vi "Set Readout Rate and EM Mode.vi"(8 "error in (no error)":errorcluster, 11 "CCDCamera in":refnum<class "CCDCamera.lvclass">) -> (0 "error out":errorcluster, 3 "CCDCamera out":refnum<class "CCDCamera.lvclass">)   [LabVIEW 2018, in "CCDCamera.lvclass"]
uses:
  CCDCamera.lvclass
  C:/Users/observer/Desktop/SPARC4_ACS/SPARC4_ACS/Simulated_CCD_Camera/Simulated_CCD_Camera.lvclass
  Simulated_CCD_Camera/Simulated_CCD_Camera.lvclass/Simulated_CCD_Camera.ctl
  Interface/Interface.lvclass/Interface.ctl
  Interface/Interface.lvclass
  Simulated_CCD_Camera/Simulated_CCD_Camera.lvclass
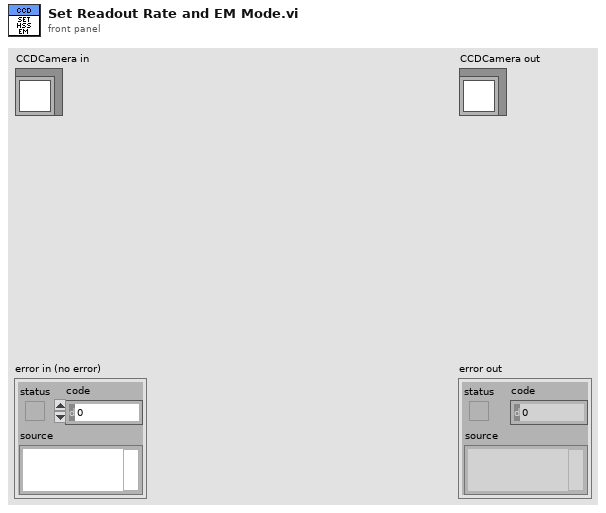
[diagram p1: front panel]
types:
  T1 = typedef "Shutter_mode typedef.ctl" = enum16{"Auto", "Open", "Close", "N/A (3)", "Open FVB Series", "Open Any Series"}
  T2 = typedef "ReadMode_mode typedef.ctl" = enum16{"Full Vertical Binning", "Multi-Track", "Random-Track", "Single-Track", "Image"}
  T3 = typedef "AcquisitionMode_mode typedef.ctl" = enum16{"Reserved (0)", "Single Scan", "Accumulate", "Kinetics", "Fast Kinetics", "Run Till Abort", "Reserved (6)", "Reserved (7)", "Reserved (8)", "Time Delayed Integration"}
  T4 = cluster{"EXPTIME":sgl, "PREAMP":enum16{"Gain 1", "Gain 2"}, "READOUT_RATE":enum16{"30 MHz", "20 MHz", "10 MHz", "1 MHz"}, "EM_GAIN":u16, "VBIN":u16, "INITIAL_LINE":u16, "INITIAL_COLUMN":u16, "FINAL_LINE":u16, "FINAL_COLUMN":u16, "#FRAMES":u32, "#CUBES":u32, "TRIGGER_MODE":enum16{"Internal", "External", "N/A", "N/A_1", "N/A_2", "N/A_3", "External Start"}, "HBIN":u16, "SHUTTER_TTL":enum16{"TTL Low", "TTL High"}, "SHUTTER_MODE":T1, "SHUTTER_OPENING_TIME":u16, "SHUTTER_CLOSING_TIME":u16, "VERTICAL_SHIFT_SPEED":u16, "READ_MODE":T2, "FRAME_TRANSFER":bool, "VERTICAL_CLOCK_VOLTAGE":enum16{"0", "+1", "+2", "+3", "+4"}, "ACQUISITION_MODE":T3, "AD_CHANNEL":u16, "EM_MODE":enum16{"Electron Multiplying", "Conventional"}, "Error In":errorcluster}
  T5 = cluster{"EXPTIME":sgl, "PREAMP":enum16{"Gain 1", "Gain 2"}, "READOUT_RATE":enum16{"30 MHz", "20 MHz", "10 MHz", "1 MHz"}, "EM_GAIN":u16, "VBIN":u16, "INITIAL_LINE":u16, "INITIAL_COLUMN":u16, "FINAL_LINE":u16, "FINAL_COLUMN":u16, "#FRAMES":u32, "#CUBES":u32, "TRIGGER_MODE":enum16{"Internal", "External", "N/A", "N/A_1", "N/A_2", "N/A_3", "External Start"}, "HBIN":u16, "SHUTTER_TTL":enum16{"TTL Low", "TTL High"}, "SHUTTER_MODE":T1, "SHUTTER_OPENING_TIME":u16, "SHUTTER_CLOSING_TIME":u16, "VERTICAL_SHIFT_SPEED":u16, "READ_MODE":T2, "FRAME_TRANSFER":bool, "VERTICAL_CLOCK_VOLTAGE":enum16{"0", "+1", "+2", "+3", "+4"}, "ACQUISITION_MODE":T3, "AD_CHANNEL":u16, "EM_MODE":enum16{"Electron Multiplying", "Conventional"}}
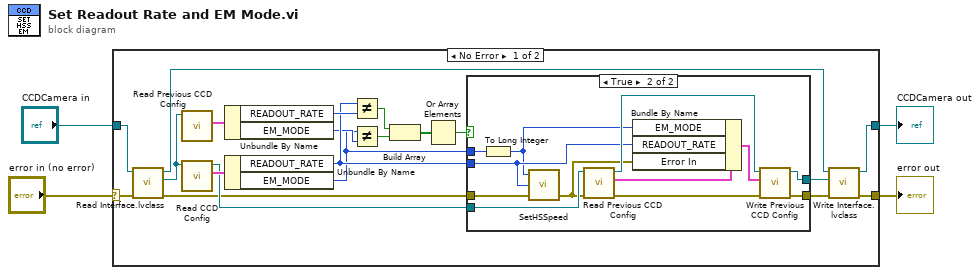
[diagram p0: block diagram]
diagram:
  n1 = case shown="No Error" "error in (no error)" {
    selector: "error in (no error)" -> [w23 w40]
    tunnel: [w13 w40] -> w2
    tunnel: [w11 w39] -> w1
    tunnel: "CCDCamera in" -> [w24 w39]
    frame No Error {
      n2 = call "Read Interface.lvclass.vi"("error in (no error)"=w23, "Simulated_CCD_Camera in"=w24) -> ("error out"=w17:errorcluster, "Interface.lvclass"=w22:refnum<class "Interface.lvclass">, "Simulated_CCD_Camera out"=w14:refnum<class "CCDCamera.lvclass">)  [unwired: 7 in]
      n3 = call "Read Previous CCD Config.vi"("Interface in"=w22) -> ("Previous CCD Config"=w20:T4)  [unwired: 8 in, 2 out]
      n4 = call "Read CCD Config.vi"("Interface in"=w22) -> ("CCD Config"=w21:T5, "Interface out"=w18:refnum<class "Interface.lvclass">)  [unwired: 8 in, 1 out]
      n5 = Unbundle By Name(w20) -> ("READOUT_RATE"=w19:enum16{"30 MHz", "20 MHz", "10 MHz", "1 MHz"}, "EM_MODE"=w10:enum16{"Electron Multiplying", "Conventional"})
      n6 = Unbundle By Name(w21) -> ("READOUT_RATE"=w12:enum16{"30 MHz", "20 MHz", "10 MHz", "1 MHz"}, "EM_MODE"=w5:enum16{"Electron Multiplying", "Conventional"})
      n7 = Not Equal?(x=w12, y=w19) -> (x != y?=w9:bool)
      n8 = Not Equal?(x=w5, y=w10) -> (x != y?=w8:bool)
      n9 = Build Array(w9, w8) -> (w7:bool[])
      n10 = Or Array Elements(Boolean array=w7) -> (logical OR=w6:bool)
      n11 = case shown="True" w6 {
        tunnel: w18 -> [w26 w38]
        tunnel: w17 -> [w25 w30]
        tunnel: [w26 w33] -> w16
        tunnel: [w25 w32] -> w15
        tunnel: w12 -> [_ w29]
        tunnel: w5 -> [_ w28]
        frame False {
        }
        frame True {
          n12 = To Long Integer(number=w28) -> (32bit integer=w27:i32)
          n13 = call <userlib>:"SetHSSpeed.vi"("error in (no error)"=w30, "index"=w29, "type"=w27) -> ("error out"=w31:errorcluster)  [unwired: 1 in, 1 out]
          n14 = call "Read Previous CCD Config.vi"("error in (no error)"=w31, "Interface in"=w38) -> ("error out"=w35:errorcluster, "Previous CCD Config"=w37:T4, "Interface out"=w34:refnum<class "Interface.lvclass">)  [unwired: 7 in]
          n15 = Bundle By Name(cluster=w37, "EM_MODE"=w27, "READOUT_RATE"=w29, "Error In"=w31) -> (w36:T4)
          n16 = call "Write Previous CCD Config.vi"("error in (no error)"=w35, "Previous CCD Config"=w36, "Interface in"=w34) -> ("error out"=w32:errorcluster, "Interface out"=w33:refnum<class "Interface.lvclass">)  [unwired: 7 in]
        }
      }
      n17 = call "Write Interface.lvclass.vi"("error in (no error)"=w15, "Interface.lvclass"=w16, "Simulated_CCD_Camera in"=w14) -> ("error out"=w13:errorcluster, "Simulated_CCD_Camera out"=w11:refnum<class "CCDCamera.lvclass">)  [unwired: 7 in]
    }
    frame Error {
    }
  }
  "error out" <- w2
  "CCDCamera out" <- w1
